vi "Save_to_Project.vi"(8 "error in (no error)":errorcluster, 9 "index in":string, 10 "buildObject":T1, 11 "Class in":refnum<class "IB_Source.lvclass">) -> (0 "error out":errorcluster, 1 "index out":string, 2 "buildObject out":T1, 3 "Class out":refnum<class "IB_Source.lvclass">, 5 "saved?":bool)   [LabVIEW 2020, in "IB_Source.lvclass"]
uses:
  <vilib>/AppBuilder/IB_Classes/Source/IB_Source.lvclass
  <vilib>/AppBuilder/IB_Classes/Source/IB_Source.lvclass/IB_Source.ctl
  <vilib>/AppBuilder/IB_RW_Project/IB_RW_Project_PropBag_Action.ctl
  <resource>/Framework/Providers/API/ItemRef.ctl
  <vilib>/AppBuilder/IB_RW_Project/IB_RW_Project_Source_Data.ctl
panel:
  in  "data":T2
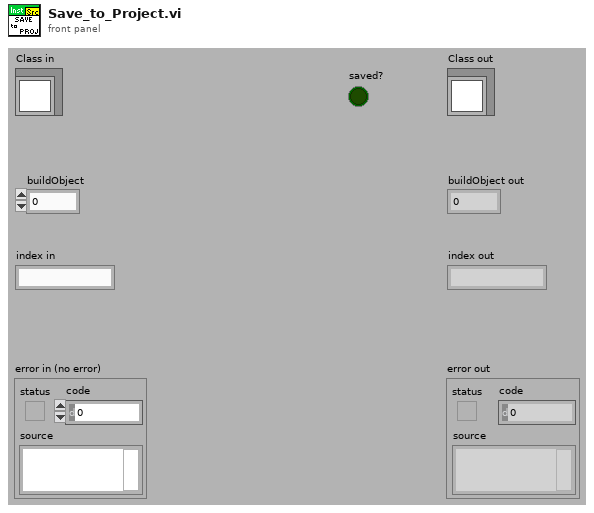
[diagram p1: front panel]
types:
  T1 = typedef "ItemRef.ctl" = u64
  T2 = typedef "IB_RW_Project_Source_Data.ctl" = cluster{"name":string, "tag":string, "dest":string, "str ref?":bool}
  T3 = typedef "IB_RW_Project_PropBag_Action.ctl" = enum16{"read", "write", "clear", "readPrevious", "writePrevious", "clearPrevious"}
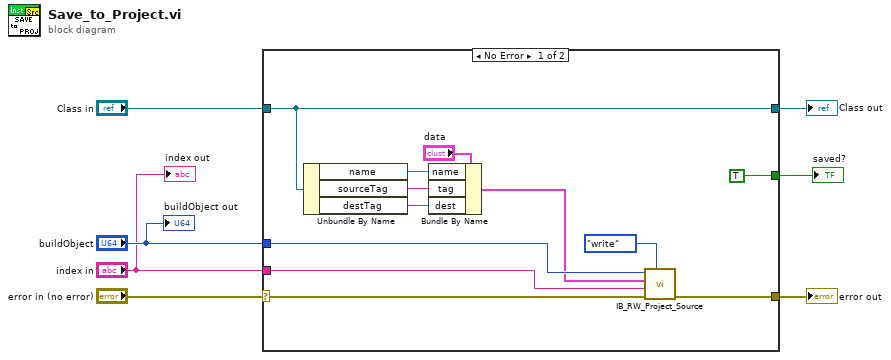
[diagram p0: block diagram]
diagram:
  n1 = case shown="No Error" "error in (no error)" {
    selector: "error in (no error)" -> [w17 w21]
    tunnel: [w16 w21] -> w6
    tunnel: [w15 w20] -> w4
    tunnel: "Class in" -> [w15 w20]
    tunnel: "buildObject" -> [w19 _]
    tunnel: "index in" -> [w18 _]
    tunnel: [TRUE _] -> w1
    frame No Error {
      n2 = Unbundle By Name(w15) -> ("name"=w11:string, "sourceTag"=w10:string, "destTag"=w9:string)
      n3 = Bundle By Name(cluster="data", "name"=w11, "tag"=w10, "dest"=w9) -> (w13:T2)
      n4 = call <vilib>:"IB_RW_Project_Source.vi"("action"=IB_RW_Project_PropBag_Action."write", "error in (no error)"=w17, "index in"=w18, "dataSource in"=w13, "buildObject"=w19) -> ("error out"=w16:errorcluster)  [unwired: 1 in, 5 out]
    }
    frame Error {
    }
  }
  "error out" <- w6
  "Class out" <- w4
  "saved?" <- w1
  "buildObject out" <- "buildObject"
  "index out" <- "index in"
